vi "emi_Is Error.vi"(14 "error in (no error)":errorcluster) -> (3 "error out":errorcluster, 8 "Is Error":bool)   [LabVIEW 2011]
doc: "Extracts teh error status from error cluster,\n \n\nSaves Diagram space at teh expence of execution speed."
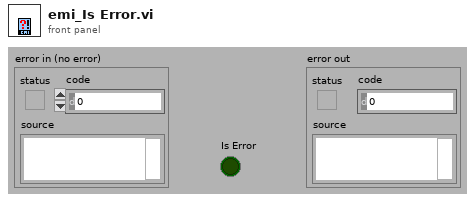
[diagram p1: front panel]
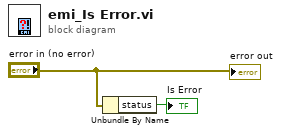
[diagram p0: block diagram]
diagram:
  n1 = Unbundle By Name("error in (no error)") -> ("status"=→"Is Error":bool)
  "error out" <- "error in (no error)"
